vi "To JSON String.vi"(0 "Display State In":T1, 5 "enable LabVIEW extensions? (T)":bool=TRUE, 7 "pretty print? (F)":bool, 9 "Container State":T2, 11 "error in (no error)":errorcluster) -> (4 "Display State Out":T1, 8 "JSON String":string, 15 "error out":errorcluster)   [LabVIEW 2017, in "Advanced Variant Tools.lvlib" / "Variant Tree.xctl"]
uses:
  Variant Tree.xctl
  <vilib>/_xctls/Container State.ctl
  State.ctl
  Advanced Variant Tools.lvlib
  <vilib>/_xctls/XControlSupport.lvlib
panel:
  # "Add Controls & Indicators that form the parameters of the method here. Hook them to the connector pane. Do not delete the controls & indicators that are already hooked to the connector pane.\n \nTo setup the parameters  for this method, right click on this item in the Project Tree & select \"Configure Method...\"."
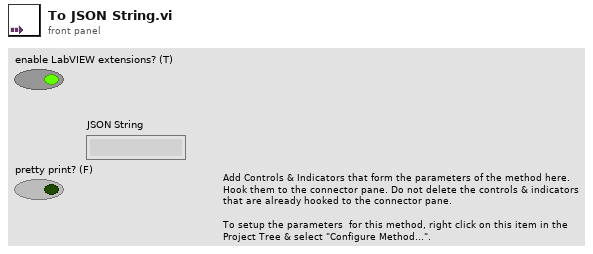
[diagram p1: front panel]
types:
  T1 = typedef "Advanced Variant Tools.lvlib/Variant Tree.xctl/State.ctl" = cluster{"Numeric":dbl}
  T2 = typedef "XControlSupport.lvlib/Container State.ctl" = cluster{"Indicator?":bool, "Run Mode?":bool, " Refnum":refnum<vi>}
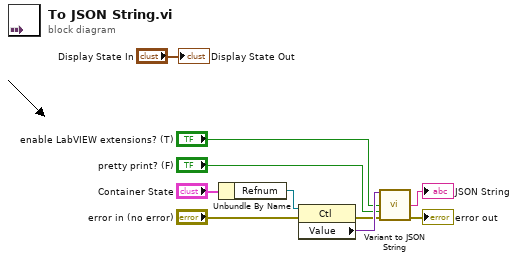
[diagram p0: block diagram]
diagram:
  n1 = Unbundle By Name("Container State") -> ("Refnum"=w8:refnum<vi>)
  n2 = property class="Ctl"(reference=w8, error in="error in (no error)") -> (error out=w5:errorcluster, "Value"=w7:variant)  [unwired: 1 out]
  n3 = call "Variant to JSON String.vi"("Variant in"=w7, "enable LabVIEW extensions? (T)"="enable LabVIEW extensions? (T)", "pretty print? (F)"="pretty print? (F)", "error in (no error)"=w5) -> ("String"=→"JSON String":string, "error out"=→"error out":errorcluster)  [unwired: 9 in, 1 out]
  "Display State Out" <- "Display State In"
